vi "Prepare Paths For Expiration Check.vi"(0 "Scalar SG Path Group in":refnum<class "SG SC2250 Path Group.lvclass">, 5 "TSM Context":T1, 11 "error in (no error)":errorcluster) -> (4 "Scalar SG Path Group out":refnum<class "SG SC2250 Path Group.lvclass">, 15 "error out":errorcluster)   [LabVIEW 2023, in "RFFixtureCharact.RFPM.lvlib" / "SG SC2250 Path Group.lvclass"]
uses:
  SG SC2250 Path Group.lvclass
  C:/srd-semi-rfcal-software/AuxTools/STSRFFixtureCharactUtility/Source/Code Modules/Common/Base Classes/Path Group/Path Group.lvclass
  <vilib>/NI_TestStand_SemiconductorModule/NI_TestStand_Semiconductor_Module.lvlibp/PinMap/General/SemiconductorModuleContext.ctl
  Paths/SG SC2250 Path/SG SC2250 Path.lvclass
  C:/srd-semi-rfcal-software/AuxTools/STSRFFixtureCharactUtility/Source/Code Modules/Common/Base Classes/Path/Path.lvclass
  C:/srd-semi-rfcal-software/AuxTools/STSRFFixtureCharactUtility/Source/Code Modules/Fixture/RFPM/Scalar/Paths/SG Path/SG 18GHz Path.lvclass
  Charact Result Accessor/Scalar/Scalar Charact Result Accessor.lvclass
  C:/srd-semi-rfcal-software/AuxTools/STSRFFixtureCharactUtility/Source/Code Modules/Fixture/RFPM/Charact Result Accessor/Base/Charact Result Accessor.lvclass
  C:/srd-semi-rfcal-software/AuxTools/STSRFFixtureCharactUtility/Source/Code Modules/Common/Result Accessor/Result Accessor.lvclass
  <vilib>/NI_TestStand_SemiconductorModule/NI_TestStand_Semiconductor_Module.lvlibp/PinMap/RF/RFmx/PinToNIRFmxSession.vi
  Common/Base Classes/Path/Path.lvclass
  Common/Result Accessor/Result Accessor.lvclass
  <vilib>/NI_TestStand_SemiconductorModule/NI_TestStand_Semiconductor_Module.lvlibp
  Common/Base Classes/Path Group/Path Group.lvclass
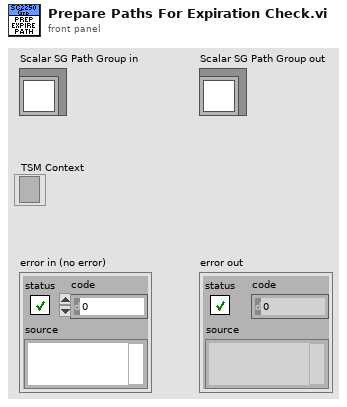
[diagram p1: front panel]
types:
  T1 = typedef "NI_TestStand_Semiconductor_Module.lvlibp/SemiconductorModuleContext.ctl" = refnum<k7>
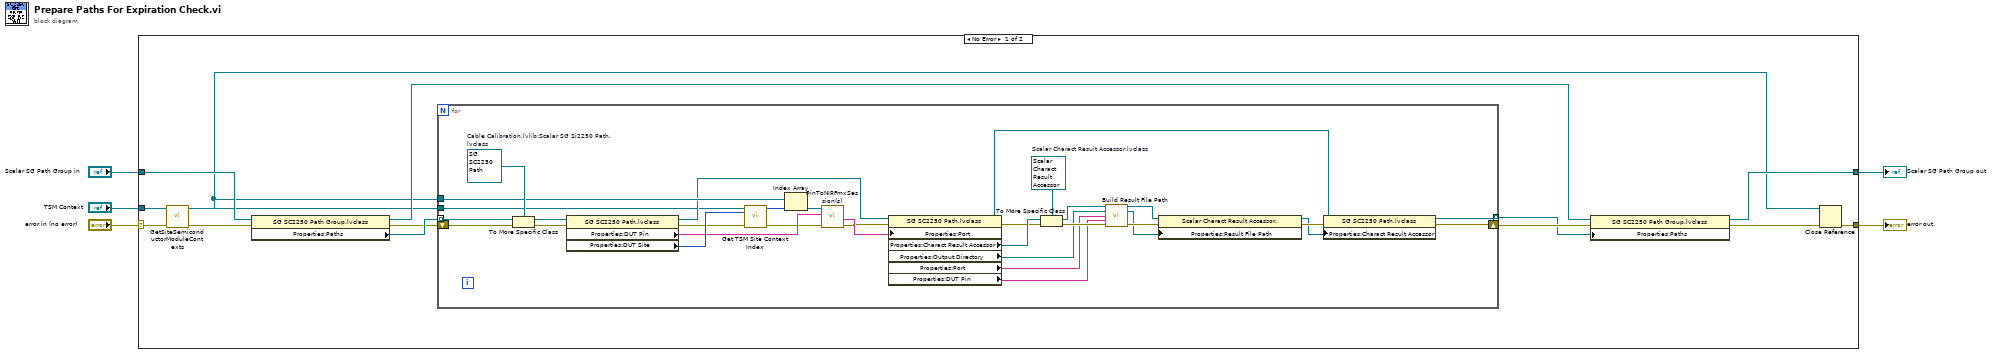
[diagram p0: block diagram]
diagram:
  n1 = case shown="No Error" "error in (no error)" {
    selector: "error in (no error)" -> [w9 w51]
    tunnel: "Scalar SG Path Group in" -> [w8 w52]
    tunnel: [w14 w52] -> w4
    tunnel: "TSM Context" -> [w7 _]
    tunnel: [w11 w51] -> w1
    frame No Error {
      n2 = call <vilib>:"GetSiteSemiconductorModuleContexts.vi"("error in (no error)"=w9, "Semiconductor Module Context"=w7) -> ("error out"=w13:errorcluster, "Site Semiconductor Module Contexts"=w6:T1[])  [unwired: 8 in]
      n3 = property class="SG SC2250 Path Group.lvclass"(reference=w8, error in=w13) -> (reference out=w15:refnum<class "SG SC2250 Path Group.lvclass">, error out=w17:errorcluster, "Properties:Paths"=w18:refnum<class "Path.lvclass">[])
      n4 = for {
        tunnel: w18 -> [w50] mode=indexing
        shift-right: [w31] -> w16
        shift-left: w17 -> [w42]
        tunnel: [w30] -> w12 mode=indexing
        tunnel: w6 -> [w47]
        tunnel: w7 -> [w19]
        w35 = refnum<class "Scalar Charact Result Accessor.lvclass"> refnum  # Scalar Charact Result Accessor.lvclass
        w48 = refnum<class "SG SC2250 Path.lvclass"> refnum  # Cable Calibration.lvlib:Scalar SG Si2250 Path.lvclass
        n5 = To More Specific Class(target class=w48, reference=w50, error in=w42) -> (specific class reference=w49:refnum<class "SG SC2250 Path.lvclass">, error out=w41:errorcluster)
        n6 = property class="SG SC2250 Path.lvclass"(reference=w49, error in=w41) -> (reference out=w36:refnum<class "SG SC2250 Path.lvclass">, error out=w38:errorcluster, "Properties:DUT Pin"=w40:string, "Properties:DUT Site"=w46:i32)
        n7 = call "Get TSM Site Context Index.vi"("Semiconductor Module Context"=w19, "Site Number"=w46, "error in (no error)"=w38) -> ("index of Site TSM Context"=w39:i32, "error out"=w37:errorcluster)  [unwired: 11 in]
        n8 = Index Array(array=w47, index=w39) -> (element=w45:T1)
        n9 = call-poly <vilib>:"PinToNIRFmxSession(s).vi"("error in (no error)"=w37, "Pin"=w40, "Semiconductor Module Context"=w45) -> ("error out"=w43:errorcluster, "Port"=w44:string)  [unwired: 4 in, 3 out]
        n10 = property class="SG SC2250 Path.lvclass"(reference=w36, error in=w43, "Properties:Port"=w44) -> (reference out=w28:refnum<class "SG SC2250 Path.lvclass">, error out=w29:errorcluster, "Properties:Charact Result Accessor"=w32:refnum<class "Result Accessor.lvclass">, "Properties:Output Directory"=w22:path, "Properties:Port"=w21:string, "Properties:DUT Pin"=w20:string)
        n11 = To More Specific Class(target class=w35, reference=w32, error in=w29) -> (specific class reference=w25:refnum<class "Scalar Charact Result Accessor.lvclass">, error out=w27:errorcluster)
        n12 = call-dynamic "Build Result File Path.vi"("Charact Result Accessor in"=w25, "Output Directory"=w22, "Port 1"=w21, "Port 2"=w20, "error in"=w27) -> ("Charact Result Accessor out"=w24:refnum<class "Scalar Charact Result Accessor.lvclass">, "Result File Path"=w23:path, "error out"=w26:errorcluster)  [unwired: 8 in]
        n13 = property class="Scalar Charact Result Accessor."(reference=w24, error in=w26, "Properties:Result File Path"=w23) -> (reference out=w33:refnum<class "Scalar Charact Result Accessor.lvclass">, error out=w34:errorcluster)
        n14 = property class="SG SC2250 Path.lvclass"(reference=w28, error in=w34, "Properties:Charact Result Accessor"=w33) -> (reference out=w30:refnum<class "SG SC2250 Path.lvclass">, error out=w31:errorcluster)
      }
      n15 = property class="SG SC2250 Path Group.lvclass"(reference=w15, error in=w16, "Properties:Paths"=w12) -> (reference out=w14:refnum<class "SG SC2250 Path Group.lvclass">, error out=w10:errorcluster)
      n16 = Close Reference(reference=w6, error in (no error)=w10) -> (error out=w11:errorcluster)
    }
    frame Error {
    }
  }
  "error out" <- w1
  "Scalar SG Path Group out" <- w4
